vi "TCP write formatter (SubVI).vi"(2 "String input":string) -> (5 "Input Length in String":string, 6 "Original string":string)   [LabVIEW 2020]
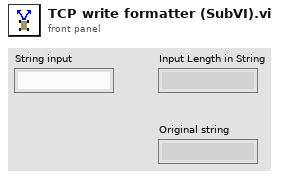
[diagram p1: front panel]
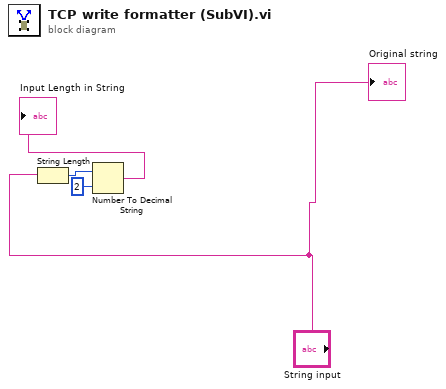
[diagram p0: block diagram]
diagram:
  n1 = String Length(string="String input") -> (length=w3:i32)
  n2 = Number To Decimal String(number=w3, width (-)=i16 2) -> (decimal integer string=→"Input Length in String":string)
  "Original string" <- "String input"
